vi "create auto tab.vi"() -> ()   [LabVIEW 2019]
uses:
  Controls/Tab Button.ctl
panel:
  out "NewVal":T1(array[cluster])
  in  "Array":T2
  in  "Add Tab":bool
  in  "stop":bool
  in  "Tab Control":enum32{"Page 1"}(tab)
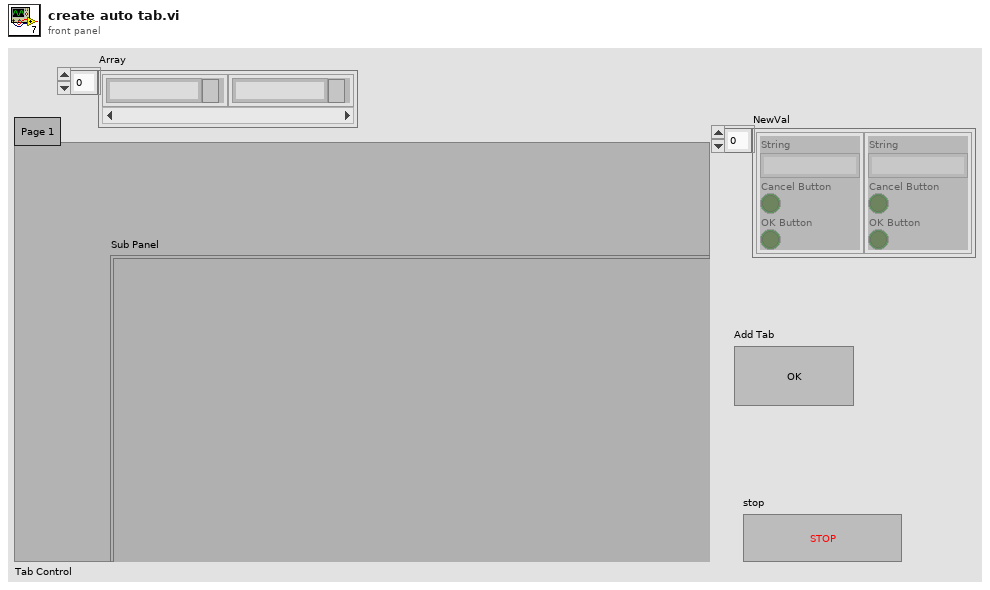
[diagram p1: front panel]
types:
  T1 = cluster{"String":string, "Cancel Button":bool, "OK Button":bool}[]
  T2 = typedef "Tab Button.ctl" = cluster{"String":string, "Cancel Button":bool, "OK Button":bool}[]
  T3 = enum32{"invalid app kind", "Development System", "Run Time System", "Student Edition", "Embedded LabVIEW", "Evaluation", "Custom"}
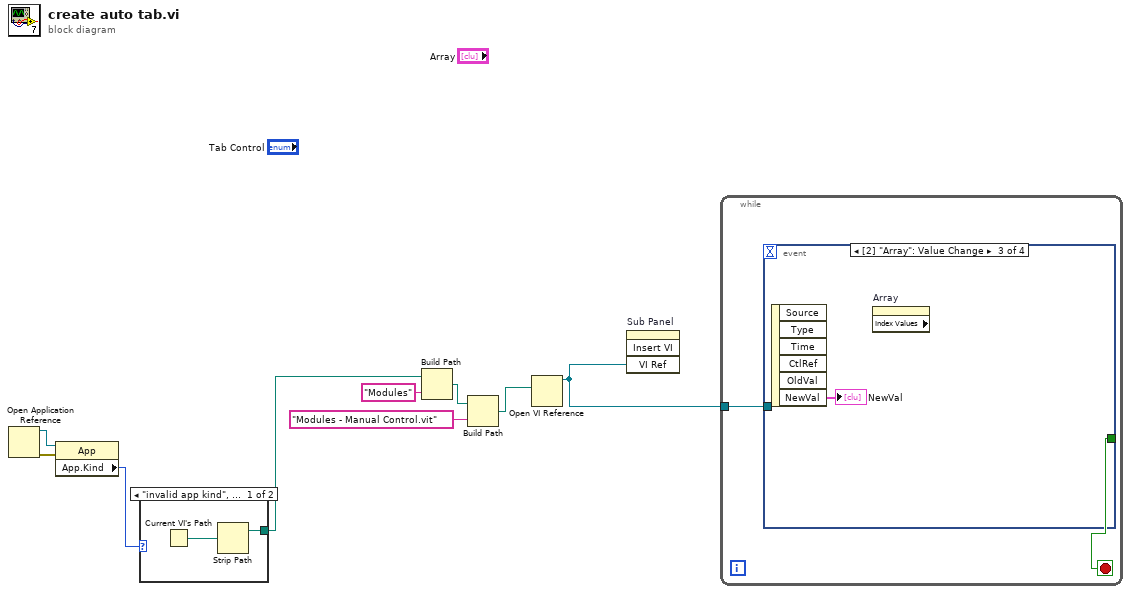
[diagram p0: block diagram]
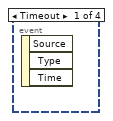
[diagram p2: hidden frame]
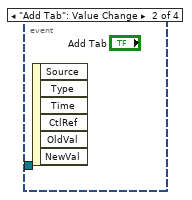
[diagram p3: hidden frame]
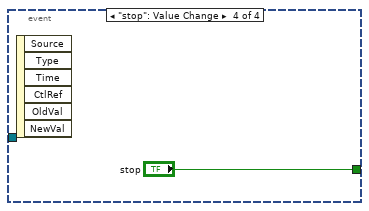
[diagram p4: hidden frame]
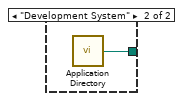
[diagram p5: hidden frame]
diagram:
  n1 = Open Application Reference() -> (0:w9:errorcluster, 3:w8:refnum<vi>)  [unwired: 4 in]
  n2 = property class="App"(reference=w8, error in=w9) -> ("App.Kind"=w7:T3)  [unwired: 2 out]
  n3 = case shown="\"invalid app kind\", Default" w7 {
    tunnel: [w10 w12] -> w3
    frame "invalid app kind", Default {
      n4 = Current VI's Path() -> (path=w11:path)
      n5 = Strip Path(path=w11) -> (stripped path=w10:path)  [unwired: 1 out]
    }
    frame "Development System" {
      n6 = call <vilib>:"Application Directory.vi"() -> ("Application Directory"=w12:path)
    }
  }
  n7 = Build Path(base path=w3, name or relative path="Modules") -> (appended path=w6:path)
  n8 = Build Path(base path=w6, name or relative path="Modules - Manual Control.vit") -> (appended path=w2:path)
  n9 = Open VI Reference(vi path=w2) -> (vi reference=w1:refnum<vi>)  [unwired: 5 in, 1 out]
  n10 = invoke on="Sub Panel" class="SubPnl" method="Insert VI"("VI Ref"=w1) -> ()  [unwired: 3 in, 4 out]
  n11 = while {
    tunnel: w1 -> [w14]
    stop <- w13 stop-if-true
    n12 = event shown="[2] \"Array\": Value Change" {
      selector: _ -> [_ _ _ _]
      dyn-events: _ -> [_ _ _ _]
      timeout: _ -> [_ _ _ _]
      tunnel: w14 -> [_ _ _ _]
      tunnel: [_ _ _ "stop"] -> w13
      event Timeout {
        n13 = event-data() -> ()  [unwired: 1 in, 3 out]
      }
      event "Add Tab": Value Change {
        n14 = event-data() -> ()  [unwired: 1 in, 6 out]
      }
      event Value Change {
        n15 = event-data() -> ("NewVal"=→"NewVal":T2)  [unwired: 1 in, 5 out]
        n16 = property on="Array" class="Arr" props=["Index Values"]() -> ()  [unwired: 2 in, 3 out]
      }
      event "stop": Value Change {
        n17 = event-data() -> ()  [unwired: 1 in, 6 out]
      }
    }
  }
